vi "CollectSensorDataGLD.vi"(11 "data (can be any type)":string) -> (1 "grams (GF)":dbl, 2 "Accel (Dyna LF)":dbl, 6 "Volt (Static LF)":dbl)   [LabVIEW 2019]
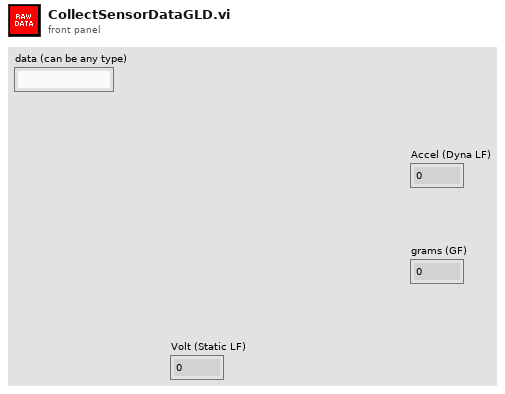
[diagram p1: front panel]
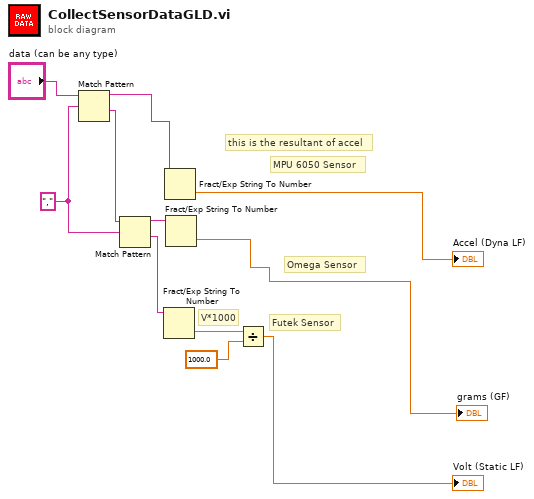
[diagram p0: block diagram]
diagram:
  w4 = ","
  # "V*1000"
  # "Futek Sensor"
  # "Omega Sensor"
  # "this is the resultant of accel"
  # "MPU 6050 Sensor"
  n1 = Match Pattern(string="data (can be any type)", regular expression=w4) -> (before substring=w3:string, after substring=w2:string)  [unwired: 1 in, 2 out]
  n2 = Match Pattern(string=w2, regular expression=w4) -> (before substring=w1:string, after substring=w5:string)  [unwired: 1 in, 2 out]
  n3 = Fract/Exp String To Number(string=w5) -> (number=w7:dbl)  [unwired: 3 in, 1 out]
  n4 = Fract/Exp String To Number(string=w3) -> (number=→"Accel (Dyna LF)":dbl)  [unwired: 3 in, 1 out]
  n5 = Fract/Exp String To Number(string=w1) -> (number=→"grams (GF)":dbl)  [unwired: 3 in, 1 out]
  n6 = Divide(x=w7, y=1000.0) -> (x/y=→"Volt (Static LF)":dbl)
